vi "G#Object_GetParent.vi"(0 "reference in":refnum<class "G#Object.lvclass">, 5 "error in (no error)":errorcluster) -> (14 "parent type ref":refnum<class "G#Object.lvclass">, 15 "parent class name":string, 16 "parent full class name":string, 17 "is base class?":bool, 19 "error out":errorcluster)   [LabVIEW 2020, in "G#Object.lvclass"]
doc: "Returns the name and type of the parent class."
uses:
  <vilib>/addons/_AddQ/G#Object/G#Object.lvclass
  <vilib>/addons/_AddQ/G#Object/utils/G#Object_State.ctl
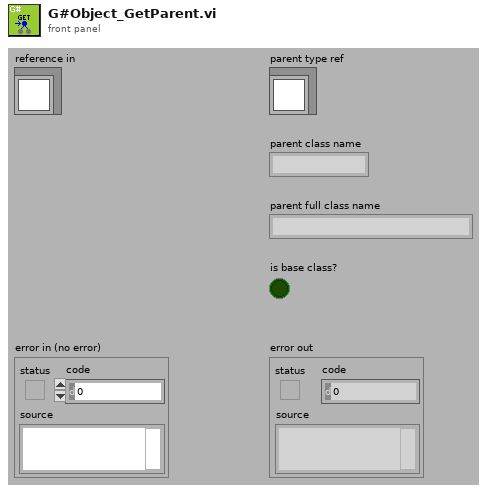
[diagram p1: front panel]
types:
  T1 = typedef "G#Object.lvclass/G#Object_State.ctl" = enum16{"Clear", "Create", "Delete", "Get class attributes", "Class hierarchy", "Get attribute value", "Set attribute value"}
  T2 = typedef "G#Object.lvclass/G#Object_ClassHierarchy.ctl" = cluster{"ClassName":string, "FullClassName":string, "ClassPath":path, "IsLeaf":bool}
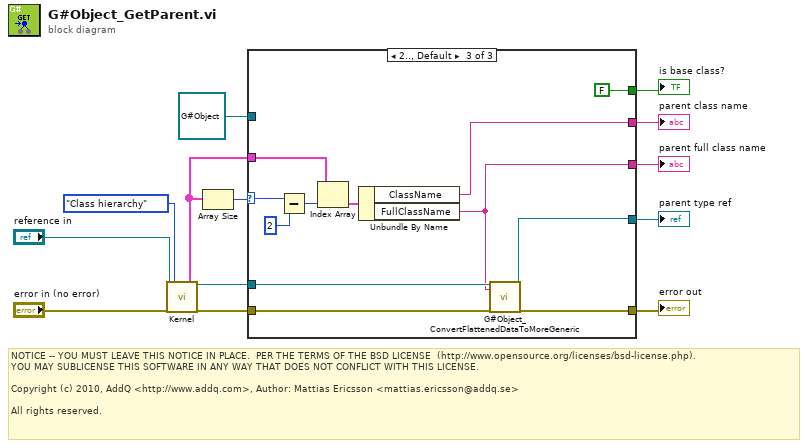
[diagram p0: block diagram]
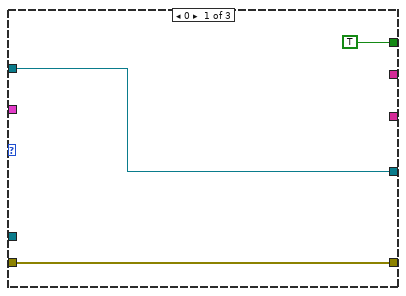
[diagram p2: hidden frame]
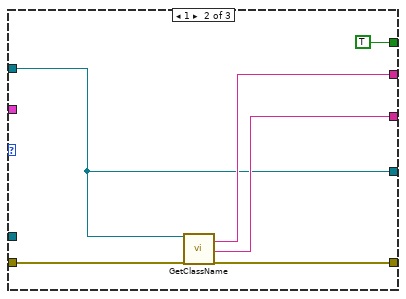
[diagram p3: hidden frame]
diagram:
  # "NOTICE -- YOU MUST LEAVE THIS NOTICE IN PLACE.  PER THE TERMS OF THE BSD LICENSE  (http://www.opensource.org/licenses/bsd-license.php).\nYOU MAY SUBLICENSE THIS SOFTWARE IN ANY WAY THAT DOES NOT CONFLICT WITH THIS LICENSE.\n\nCopyright (c) 2010, AddQ <http://www.addq.com>, Author: Mattias Ericsson <mattias.ericsson@addq.se>\n\nAll rights reserved."
  n1 = call-dynamic "Kernel.vi"("reference in"="reference in", "error in (no error)"="error in (no error)", "state"=G#Object_State."Class hierarchy") -> ("class hierarchy"=w11:T2[], "reference out"=w1:refnum<class "G#Object.lvclass">, "error out"=w8:errorcluster)  [unwired: 8 in, 6 out]
  n2 = Array Size(array=w11) -> (size(s)=w5:i32)
  n3 = case shown="2.., Default" w5 {
    selector: w5 -> [_ _ w29]
    tunnel: w11 -> [_ _ w32]
    tunnel: [_ w20 w30] -> w10
    tunnel: [_ w19 w24] -> w9
    tunnel: w8 -> [w16 w22 w27]
    tunnel: [w16 w21 w26] -> w7
    tunnel: [w14 w18 w23] -> w6
    tunnel: [TRUE TRUE FALSE] -> w3
    tunnel: refnum<class "G#Object.lvclass"> refnum ("reference in") -> [w14 w18 _]
    tunnel: w1 -> [_ _ w25]
    frame 0 {
    }
    frame 1 {
      n4 = call-dynamic "GetClassName.vi"("reference in"=w18, "error in (no error)"=w22) -> ("class name"=w20:string, "full class name"=w19:string, "error out"=w21:errorcluster)  [unwired: 13 in, 2 out]
    }
    frame 2.., Default {
      n5 = Subtract(x=w29, y=2) -> (x-y=w33:i32)
      n6 = Index Array(array=w32, index=w33) -> (element=w31:T2)
      n7 = Unbundle By Name(w31) -> ("ClassName"=w30:string, "FullClassName"=w24:string)
      n8 = call <vilib>:"G#Object_ConvertFlattenedDataToMoreGeneric.vi"("reference in"=w25, "full class name"=w24, "error in (no error)"=w27) -> ("reference converterrd"=w23:refnum<class "G#Object.lvclass">, "error out"=w26:errorcluster)  [unwired: 15 in]
    }
  }
  "error out" <- w7
  "parent type ref" <- w6
  "parent class name" <- w10
  "parent full class name" <- w9
  "is base class?" <- w3
